vi "SMTP Email Format Text Message.vi"(5 "translit":string, 6 "character set":string, 7 "last chunk (T)":bool=TRUE, 8 "prev data (\"\")":string, 9 "text":string) -> (0 "real charset":string, 2 "next data":string, 3 "formated text":string)   [LabVIEW 2011, in "NewNI_SMTPEmail.lvlib"]
doc: "This VI takes a text message (or a chunk of it) and makes it MIME compliant so that it can be sent over the net using SMTP protocol. The VI uses quoted-printable encoding for the extended character set. The parameter Last Chunk is used when a large amount of data has to be sent (for example we are reading data from a file). In this case we can convert the data in chunks. However, in order for the VI to correctly assemble the pieces it has to keep the state of the chunks. So when the last chunk of the same data is sent, the Last Chunk parameter must be set to True."
uses:
  NewNI_SMTPEmail.lvlib
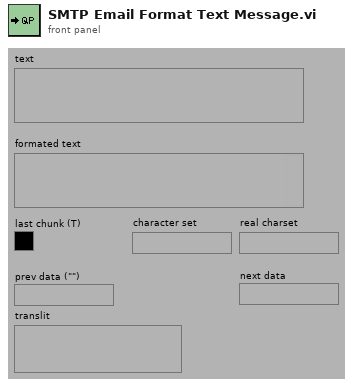
[diagram p1: front panel]
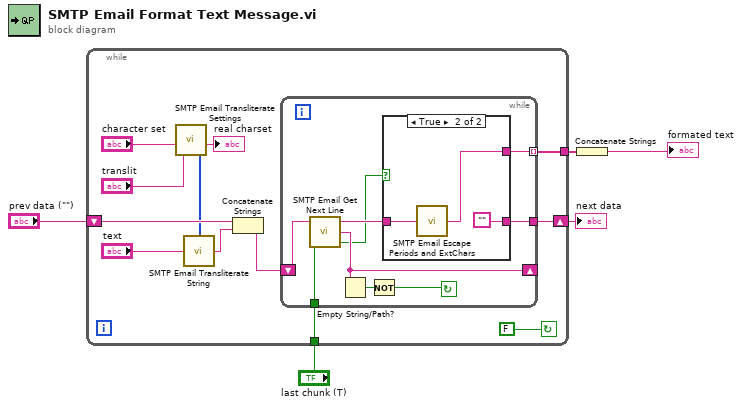
[diagram p0: block diagram]
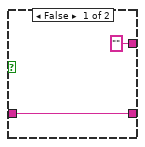
[diagram p2: hidden frame]
diagram:
  n1 = while {
    tunnel: "last chunk (T)" -> [w8]
    tunnel: [w9] -> w5
    shift-left: "prev data (\"\")" -> [w15]
    shift-right: [w16] -> w3
    stop <- FALSE continue-if-true
    n2 = call "SMTP Email Transliterate Settings.vi"("transliteration"="translit", "character set"="character set") -> ("map"=w14:u8[], "charset out"=→"real charset":string)  [unwired: 4 out]
    n3 = call "SMTP Email Transliterate String.vi"("text in"="text", "map"=w14) -> ("text out"=w13:string)
    n4 = Concatenate Strings(w15, w13) -> (w17:string)
    n5 = while {
      tunnel: w8 -> [w18]
      tunnel: [w25] -> w9 mode=indexing
      shift-left: w17 -> [w20]
      shift-right: [w23] -> _
      tunnel: [w26] -> w16
      stop <- w21 continue-if-true
      n6 = call "SMTP Email Get Next Line.vi"("last chunk"=w18, "string"=w20) -> ("found eoln"=w19:bool, "after eoln"=w23:string, "before eoln"=w24:string)  [unwired: 1 in]
      n7 = Empty String/Path?(string/path=w23) -> (empty?=w22:bool)
      n8 = Not(x=w22) -> (.not. x?=w21:bool)
      n9 = case shown="True" w19 {
        tunnel: ["" ("Formatted Line of Text") w29] -> w25
        tunnel: w24 -> [w28 w30]
        tunnel: [w28 ""] -> w26
        frame False {
        }
        frame True {
          n10 = call "SMTP Email Escape Periods and ExtChars.vi"("string"=w30) -> ("quoted string"=w29:string)
        }
      }
    }
  }
  "next data" <- w3
  n11 = Concatenate Strings(w5) -> (→"formated text":string)
